vi "Stop Core.vi"(10 "final error code":i32 caption="最终错误代码", 11 "Dialogue in":refnum<class "Dialogue.lvclass"> caption="操作者输入") -> (3 "Dialogue out":refnum<class "Dialogue.lvclass"> caption="操作者输出")   [LabVIEW 2014, in "Dialogue.lvlib" / "Dialogue.lvclass"]
doc: "(<B>文件名</B>：Actor Framework.lvlib:Actor.lvclass:Stop Core.vi)\n\n定义停止前操作者的动作。使用<B>最终错误代码</B>输入判断操作者是否在出错时关闭。\n\n默认情况下，该方法不执行任何动作。子孙类重写该方法，定义出错时的操作，例如，关闭操作者核心方法初始的进程。"
uses:
  Dialogue.lvclass
  Dialogue.lvclass/Dialogue.ctl
  <vilib>/ActorFramework/Actor/Actor.lvclass
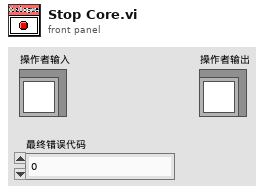
[diagram p1: front panel]
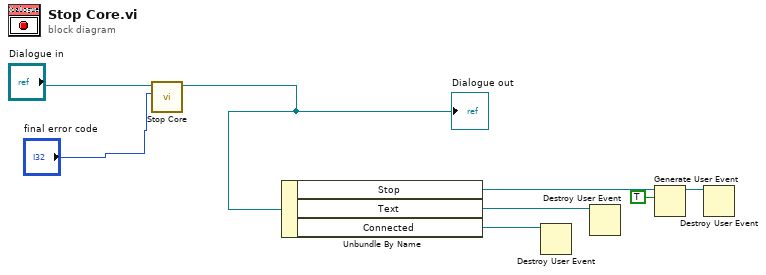
[diagram p0: block diagram]
diagram:
  n1 = call-parent "Stop Core.vi"("final error code"="final error code", "Actor in"="Dialogue in") -> ("Actor out"=w1:refnum<class "Dialogue.lvclass">)  [unwired: 9 in]
  "Dialogue out" <- w1
  n2 = Unbundle By Name(w1) -> ("Stop"=w8:refnum<user-event>, "Text"=w6:refnum<user-event>, "Connected"=w4:refnum<user-event>)
  n3 = Destroy User Event(user event=w4) -> ()  [unwired: 1 in, 1 out]
  n4 = Destroy User Event(user event=w6) -> ()  [unwired: 1 in, 1 out]
  n5 = Generate User Event(user event=w8, event data cluster=TRUE ("event data")) -> (user event out=w5:refnum<user-event>)  [unwired: 2 in, 1 out]
  n6 = Destroy User Event(user event=w5) -> ()  [unwired: 1 in, 1 out]
